vi "Write iaa.vi"(8 "error in (no error)":errorcluster, 10 "iaa":dbl[unit] min=0.0 max=6.283185307179586, 11 "RotOffset in":refnum<class "RotOffset.lvclass">) -> (0 "error out":errorcluster, 3 "RotOffset out":refnum<class "RotOffset.lvclass">)   [LabVIEW 2022 SP3, in "TCSDataDefinitions.lvlib" / "TCSCommand.lvlib" / "OffsetCommands.lvlib" / "RotOffset.lvclass"]
uses:
  RotOffset.lvclass
  RotOffset.lvclass/RotOffset.ctl
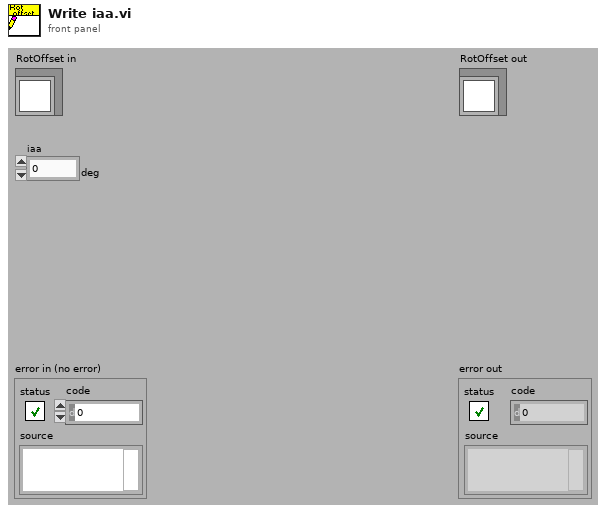
[diagram p1: front panel]
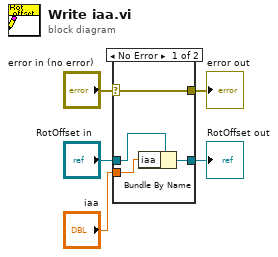
[diagram p0: block diagram]
diagram:
  n1 = case shown="No Error" "error in (no error)" {
    selector: "error in (no error)" -> [w9 w10]
    tunnel: [w9 w10] -> w4
    tunnel: [w7 w11] -> w2
    tunnel: "RotOffset in" -> [w8 w11]
    tunnel: "iaa" -> [w6 _]
    frame No Error {
      n2 = Bundle By Name(cluster=w8, "iaa"=w6) -> (w7:refnum<class "RotOffset.lvclass">)
    }
    frame Error {
    }
  }
  "error out" <- w4
  "RotOffset out" <- w2
